vi "CPP_AeroProbePtByPt.vi"(1 "Data":dbl[][](array[numeric])=array820x5[4100 elements], 3 "Old5HoleProbe?":bool, 5 "Calibration Folder Path":path=path "G:/5HoleProbe", 9 "Zeroes":dbl[](array[numeric])=[28.058802677606455, 27.889044978558935, 28.67367725910595, 28.022419773131148, 29.113875113378995], 11 "Graphs":bool=TRUE, 12 "Pressure (torr)":dbl=629.1373350315, 13 "Temperature (K)":dbl=298.4017) -> (4 "VmagUVWCone":dbl[][](array[numeric]), 6 "TotalPoints":i32, 10 "Plug in titles":string[](array[string])=["Good", "AllNegative", "dPTooSmall", "P1smallest", "FailedToReduce", "ExceedMaxCone", "U.LT.0"], 15 "errors":i16[](array[numeric]))   [LabVIEW 2013]
uses:
  CPP_Aeroprobe/VWflipperScalar.vi
panel:
  out "Progress":dbl(slide)=819.0 max=820.0 scale=-1.0..820.0
  # "1\n\n\n2\n\n\n4\n\n\n8\n\n16\n\n\n32\n\n\n64"
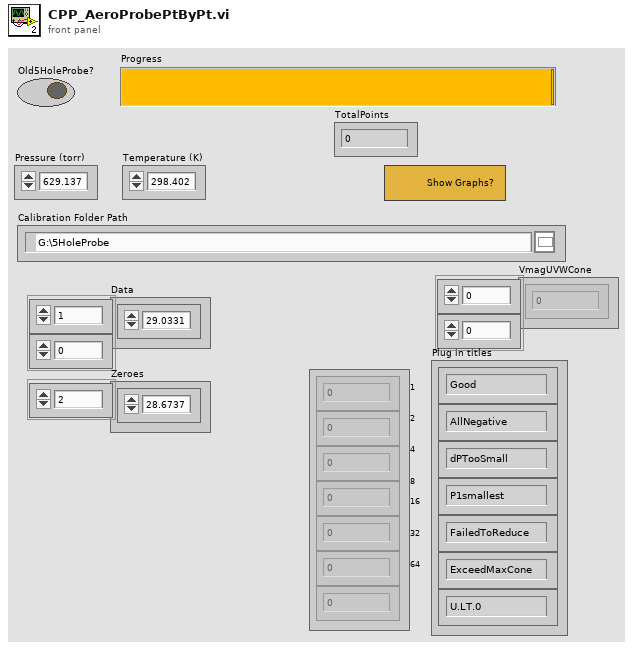
[diagram p1: front panel]
types:
  T1 = cluster{"[0]":dbl, "[1]":dbl, "[2]":dbl, "[3]":dbl, "[4]":dbl}
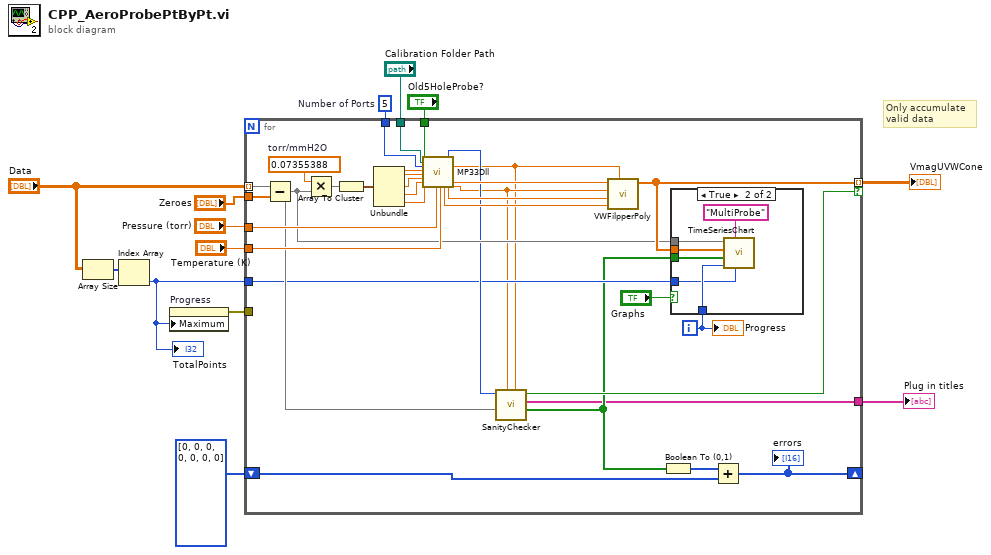
[diagram p0: block diagram]
diagram:
  w10 = 5  # Number of Ports
  # "Only accumulate\nvalid data"
  n1 = Array Size(array="Data") -> (size(s)=w6:i32[])
  n2 = Index Array(array=w6) -> (element=w2:i32)  [unwired: 1 in]
  "TotalPoints" <- w2
  n3 = property on="Progress" class="Slide (strict)"("Maximum"=w2) -> (error out=w7:errorcluster)  [unwired: 2 in, 1 out]
  n4 = for {
    tunnel: "Data" -> [w37] mode=indexing
    tunnel: "Zeroes" -> [w36]
    tunnel: [w27] -> w4 mode=indexing if=w16
    tunnel: "Calibration Folder Path" -> [w35]
    tunnel: w10 -> [w34]
    tunnel: "Old5HoleProbe?" -> [w33]
    tunnel: "Temperature (K)" -> [w32]
    tunnel: "Pressure (torr)" -> [w31]
    tunnel: w7 -> [_]
    shift-right: [w21] -> _
    shift-left: i16[] [0, 0, 0, 0, 0, 0, 0] -> [w22]
    tunnel: w2 -> [w20]
    tunnel: [w14] -> w1
    i -> [w24]
    w45 = 0.07355388  # torr/mmH2O
    n5 = Subtract(x=w37, y=w36) -> (x-y=w25:dbl[])
    n6 = Multiply(x=w45, y=w25) -> (x*y=w44:dbl[])
    n7 = Array To Cluster(array=w44) -> (cluster=w43:T1)
    n8 = Unbundle(w43) -> ("[0]"=w42:dbl, "[1]"=w41:dbl, "[2]"=w40:dbl, "[3]"=w39:dbl, "[4]"=w38:dbl)
    n9 = call "MP33Dll.vi"("Old5HoleProbe?"=w33, "Calibration Folder Path"=w35, "Number of Ports"=w34, "P1 Torr"=w42, "P2 Torr"=w41, "P3 Torr"=w40, "P4 Torr"=w39, "P5 Torr"=w38, "Pref Torr"=w31, "TTot Kelvin"=w32) -> ("w m/s"=w28:dbl, "return type"=w23:i32, "v m/s"=w29:dbl, "Theta Degree"=w17:dbl, "VMagn m/s"=w30:dbl, "u  m/s"=w18:dbl)  [unwired: 7 in, 5 out]
    n10 = call "SanityChecker.vi"("Theta"=w17, "U"=w18, "ZeroedPressures"=w25, "ReductionError"=w23) -> ("ErrorArray"=w15:bool[], "Plug in titles"=w14:string[], "CleanPoint"=w16:bool)  [unwired: 5 in]
    n11 = call-poly "VWFilpperPoly.vi"("Theta Degree"=w17, "Probe w m/s"=w28, "Probe v m/s"=w29, "Probe u  m/s"=w18, "VMagn m/s"=w30) -> ("VmagUVWCone"=w27:dbl[])  [unwired: 6 in]
    n12 = Boolean To (0,1)(Boolean=w15) -> (0, 1=w19:i16[])
    n13 = case shown="True" "Graphs" {
      tunnel: w24 -> [_ w51]
      tunnel: w25 -> [_ w50]
      tunnel: w27 -> [_ w49]
      tunnel: w15 -> [_ w48]
      tunnel: w20 -> [_ w47]
      frame False {
      }
      frame True {
        n14 = call "TimeSeriesChart.vi"("IncomingLength"=w47, "String"="MultiProbe", "iStep"=w51, "errors"=w48, "VmagUVWCone"=w49, "netPressures"=w50) -> ()  [unwired: 6 in]
      }
    }
    n15 = Add(x=w19, y=w22) -> (x+y=w21:i16[])
    "errors" <- w21
    "Progress" <- w24
  }
  "VmagUVWCone" <- w4
  "Plug in titles" <- w1
